vi "DI Error Message.vi"(11 "Faults":bool[](array[boolean])) -> (3 "Error Message":string)   [LabVIEW 2017]
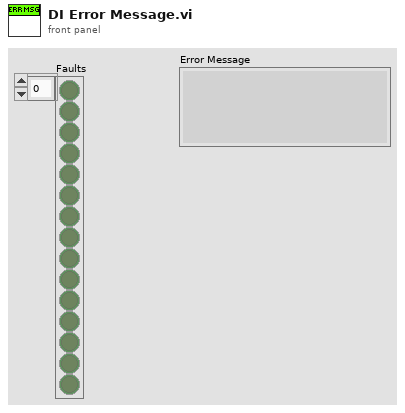
[diagram p1: front panel]
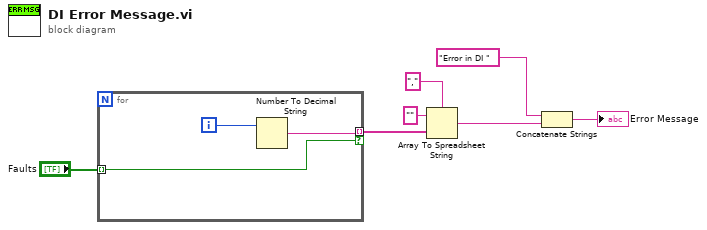
[diagram p0: block diagram]
diagram:
  n1 = for {
    tunnel: "Faults" -> [w8] mode=indexing
    tunnel: [w9] -> w6 mode=indexing if=w8
    i -> [w10]
    n2 = Number To Decimal String(number=w10) -> (decimal integer string=w9:string)  [unwired: 1 in]
  }
  n3 = Array To Spreadsheet String(delimiter (Tab)=",", array=w6, 3:"" ("format string")) -> (spreadsheet string=w3:string)
  n4 = Concatenate Strings("Error in DI " ("string"), w3) -> (→"Error Message":string)
